vi "ReadLimits.vi"(8 "error in (no error)":errorcluster, 11 "PMUConfig":T1={"Class"="M", "Fs"=50.0, "F0"=50.0}) -> (0 "error out":errorcluster, 3 "Limits":dbl[][](array[numeric])=[[1.0, 1.0, 1.0, 1.0, 1.0, 1.0, 1.0, 1.0, 0.005, 0.1], [1.0, 1.0, 1.0, 1.0, 1.0, 1.0, 1.0, 1.0, inf, inf], [1.0, 1.0, 1.0, 1.0, 1.0, 1.0, 1.0, 1.0, 0.025, inf], [1.3, 1.3, 1.3, 1.3, 1.3, 1.3, 1.3, 1.3, 0.01, inf], [1.0, 1.0, 1.0, 1.0, 1.0, 1.0, 1.0, 1.0, 0.01, 0.2], [1.0, 1.0, 1.0, 1.0, 1.0, 1.0, 1.0, 1.0, 0.01, 0.2], [3.0, 3.0, 3.0, 3.0, 3.0, 3.0, 3.0, 3.0, 0.3, 14.0], [3.0, 3.0, 3.0, 3.0, 3.0, 3.0, 3.0, 3.0, 0.3, 14.0], [0.14, 0.14, 0.14, 0.14, 0.14, 0.14, 0.14, 0.14, 0.28, 0.28], [0.005, 0.005, 0.005, 0.005, 0.005, 0.005, 0.005, 0.005, inf, inf], [0.1, 0.1, 0.1, 0.1, 0.1, 0.1, 0.1, 0.1, inf, inf], [0.14, 0.14, 0.14, 0.14, 0.14, 0.14, 0.14, 0.14, 0.28, 0.28], [0.005, 0.005, 0.005, 0.005, 0.005, 0.005, 0.005, 0.005, inf, inf], [inf, inf, inf, inf, inf, inf, inf, inf, inf, inf]])   [LabVIEW 2014]
uses:
  typedef/PMUConfig.ctl
  typedef/ctlLimits.ctl
  typedef/clRptSS.ctl
  typedef/clTveFeRFe.ctl
  typedef/clRptRamp.ctl
  typedef/clRptMod.ctl
  typedef/clRptStep.ctl
  typedef/clStepVals.ctl
  <vilib>/Utility/xml.llb/Read From XML File(string).vi
panel:
  # "VA TVE"
  # "VB TVE"
  # "VC TVE"
  # "V+ TVE"
  # "IA TVE"
  # "IB TVE"
  # "IC TVE"
  # "I+ TVE"
  # "FE"
  # "RFE"
  # "FreqRng"
  # "MagRng"
  # "Harm"
  # "OOB"
  # "Phase Mod"
  # "Ampl Mod"
  # "Ramp +"
  # "Ramp -"
  # "Phase Step Response Time"
  # "Phase Step Delay Time"
  # "Phase Step Overshoot"
  # "Mag Step Response Time"
  # "Mag Step Delay Time"
  # "Mag Step Overshoot"
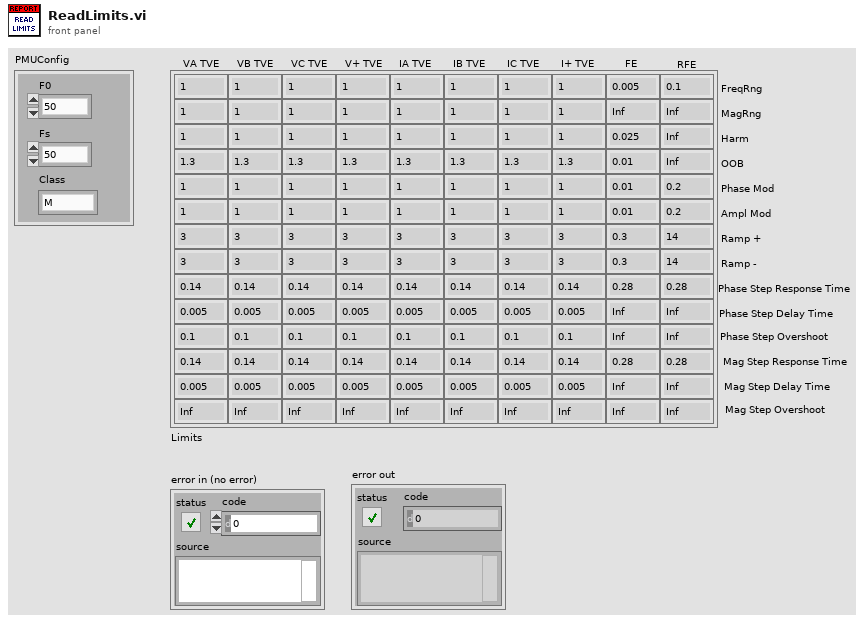
[diagram p1: front panel]
types:
  T1 = typedef "PMUConfig.ctl" = cluster{"Class":string, "Fs":dbl, "F0":dbl}
  T2 = typedef "ctlLimits.ctl" = cluster{"SteadyState":T3, "Ramp":T5, "Modulation":T6, "Step":T7, "Latency Test Limits":cluster{"Latency Limits":cluster{"Min Latency limit":dbl, "Max Latency limit":dbl}}}
  T3 = typedef "clRptSS.ctl" = cluster{"FreqResp":T4, "Harmonics":T4, "InterHarmonics":T4, "Mag":T4}
  T4 = typedef "clTveFeRFe.ctl" = cluster{"TVE":dbl, "Fe":dbl, "RFe":dbl}
  T5 = typedef "clRptRamp.ctl" = cluster{"ramp":T4}
  T6 = typedef "clRptMod.ctl" = cluster{"Phase":T4, "Amplitude":T4, "Combined":T4}
  T7 = typedef "clRptStep.ctl" = cluster{"Phase":T8, "Amplitude":T8}
  T8 = typedef "clStepVals.ctl" = cluster{"PhasorRespTime":dbl, "PhasorDelayTime":dbl, "PhaseOvershoot":dbl, "FreqRespTime":dbl, "ROCOFRespTime":dbl, "FreqOverShoot":dbl, "ROCOFOvershoot":dbl, "AmplOvershoot":dbl}
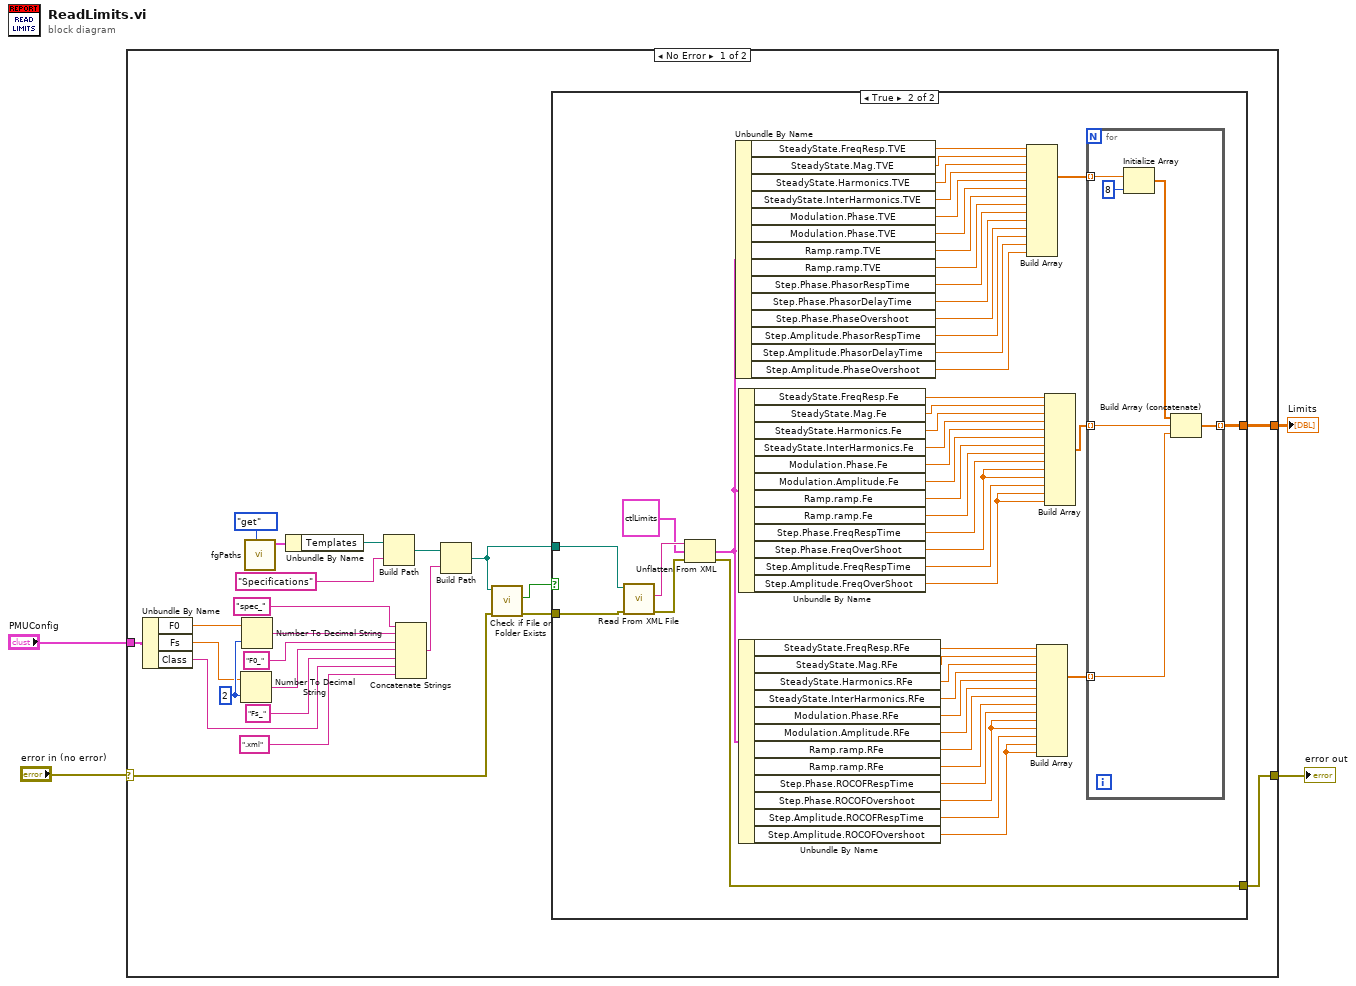
[diagram p0: block diagram]
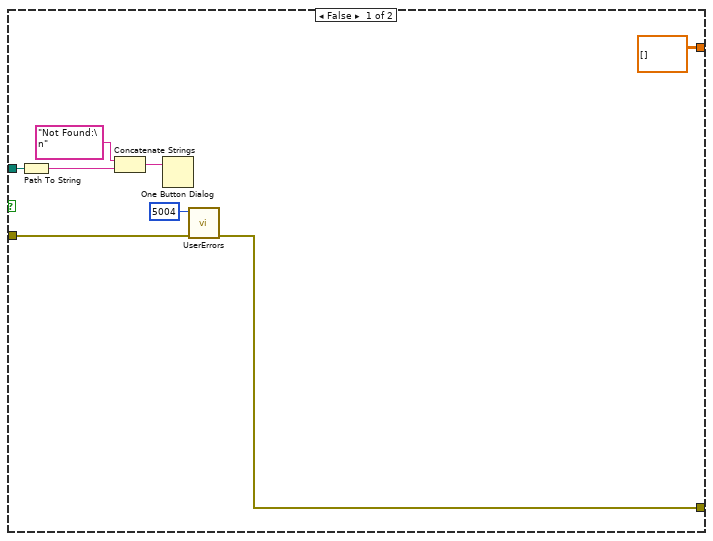
[diagram p2: hidden frame]
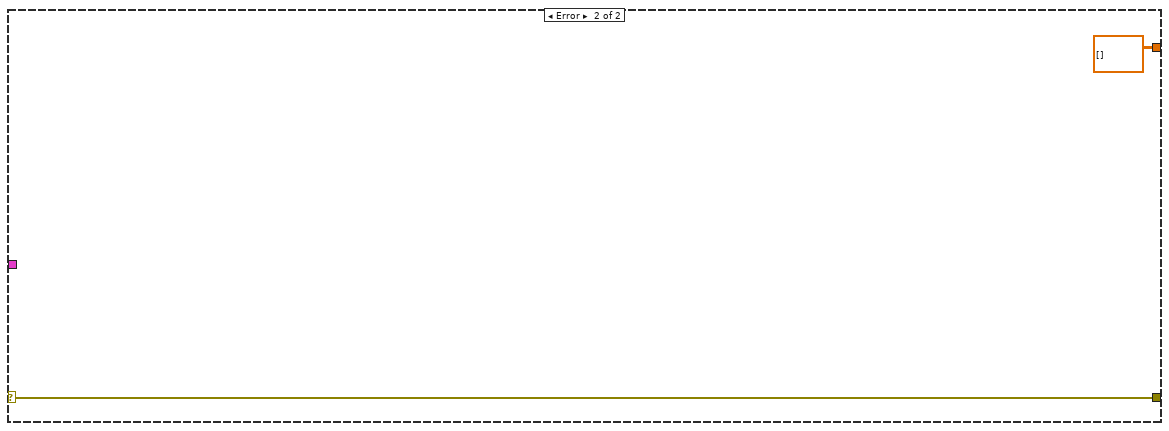
[diagram p3: hidden frame]
diagram:
  n1 = case shown="No Error" "error in (no error)" {
    selector: "error in (no error)" -> [w15 w92]
    tunnel: [w8 w92] -> w3
    tunnel: "PMUConfig" -> [w27 _]
    tunnel: [w9 dbl[][] []] -> w1
    frame No Error {
      w26 = i16 2 ("width (-)")
      n2 = Unbundle By Name(w27) -> ("F0"=w25:dbl, "Fs"=w24:dbl, "Class"=w11:string)
      n3 = Number To Decimal String(number=w24, width (-)=w26) -> (decimal integer string=w20:string)
      n4 = Number To Decimal String(number=w25, width (-)=w26) -> (decimal integer string=w22:string)
      n5 = call "fgPaths.vi"("cmd"=enum16{"init", "set", "get"}."get") -> ("clPaths"=w6:cluster{"Templates":path, "Reports":path})  [unwired: 9 in, 1 out]
      n6 = Unbundle By Name(w6) -> ("Templates"=w5:path)
      n7 = Build Path(base path=w5, name or relative path="Specifications") -> (appended path=w16:path)
      n8 = Concatenate Strings("spec_", w22, "F0_", w20, "Fs_", w11, ".xml") -> (w17:string)
      n9 = Build Path(base path=w16, name or relative path=w17) -> (appended path=w13:path)
      n10 = call <vilib>:"Check if File or Folder Exists.vi"("error in (no error)"=w15, "path"=w13) -> ("error out"=w14:errorcluster, "file or folder exists?"=w10:bool)  [unwired: 7 in, 1 out]
      n11 = case shown="True" w10 {
        tunnel: w14 -> [w35 w84]
        tunnel: w13 -> [w30 w83]
        tunnel: [w34 w50] -> w8
        tunnel: [dbl[][] [] w51] -> w9
        frame False {
          n12 = Path To String(path=w30) -> (string=w29:string)
          n13 = Concatenate Strings("Not Found:\n", w29) -> (w28:string)
          n14 = One Button Dialog(message=w28) -> ()  [unwired: 1 in, 1 out]
          n15 = call "UserErrors.vi"("error in (no error)"=w35, "[error code] (0)"=5004) -> ("error out"=w34:errorcluster)  [unwired: 9 in]
        }
        frame True {
          n16 = call-poly <vilib>:"Read From XML File.vi"("error in (no error)"=w84, "XML File Path"=w83) -> ("error out"=w81:errorcluster, "XML Elements"=w82:string)  [unwired: 7 in, 1 out]
          n17 = Unflatten From XML(xml string=w82, type=T2 {"SteadyState"={"FreqResp"={"TVE"=-inf, "Fe"=-inf, "RFe"=-inf}, "Harmonics"={"TVE"=-inf, "Fe"=-inf, "RFe"=-inf}, "InterHarmonics"={"TVE"=-inf, "Fe"=-inf, "RFe"=-inf}, "Mag"={"TVE"=-inf, "Fe"=-inf, "RFe"=-inf}}, "Ramp"={"ramp"={"TVE"=-inf, "Fe"=-inf, "RFe"=-inf}}, "Modulation"={"Phase"={"TVE"=-inf, "Fe"=-inf, "RFe"=-inf}, "Amplitude"={"TVE"=-inf, "Fe"=-inf, "RFe"=-inf}, "Combined"={"TVE"=-inf, "Fe"=-inf, "RFe"=-inf}}, "Step"={"Phase"={"PhasorRespTime"=-inf, "PhasorDelayTime"=-inf, "PhaseOvershoot"=-inf, "FreqRespTime"=-inf, "ROCOFRespTime"=-inf, "FreqOverShoot"=-inf, "ROCOFOvershoot"=-inf, "AmplOvershoot"=-inf}, "Amplitude"={"PhasorRespTime"=-inf, "PhasorDelayTime"=-inf, "PhaseOvershoot"=-inf, "FreqRespTime"=-inf, "ROCOFRespTime"=-inf, "FreqOverShoot"=-inf, "ROCOFOvershoot"=-inf, "AmplOvershoot"=-inf}}, "Latency Test Limits"={"Latency Limits"={"Min Latency limit"=0.0, "Max Latency limit"=0.0}}} ("ctlLimits"), error in (no error)=w81) -> (value=w61:T2, error out=w50:errorcluster)
          n18 = Unbundle By Name(w61) -> ("SteadyState.FreqResp.TVE"=w79:dbl, "SteadyState.Mag.TVE"=w78:dbl, "SteadyState.Harmonics.TVE"=w77:dbl, "SteadyState.InterHarmonics.TVE"=w76:dbl, "Modulation.Phase.TVE"=w75:dbl, "Modulation.Phase.TVE"=w74:dbl, "Ramp.ramp.TVE"=w73:dbl, "Ramp.ramp.TVE"=w71:dbl, "Step.Phase.PhasorRespTime"=w49:dbl, "Step.Phase.PhasorDelayTime"=w48:dbl, "Step.Phase.PhaseOvershoot"=w47:dbl, "Step.Amplitude.PhasorRespTime"=w46:dbl, "Step.Amplitude.PhasorDelayTime"=w45:dbl, "Step.Amplitude.PhaseOvershoot"=w44:dbl)
          n19 = Unbundle By Name(w61) -> ("SteadyState.FreqResp.Fe"=w70:dbl, "SteadyState.Mag.Fe"=w69:dbl, "SteadyState.Harmonics.Fe"=w68:dbl, "SteadyState.InterHarmonics.Fe"=w67:dbl, "Modulation.Phase.Fe"=w66:dbl, "Modulation.Amplitude.Fe"=w65:dbl, "Ramp.ramp.Fe"=w64:dbl, "Ramp.ramp.Fe"=w63:dbl, "Step.Phase.FreqRespTime"=w39:dbl, "Step.Phase.FreqOverShoot"=w38:dbl, "Step.Amplitude.FreqRespTime"=w37:dbl, "Step.Amplitude.FreqOverShoot"=w36:dbl)
          n20 = Unbundle By Name(w61) -> ("SteadyState.FreqResp.RFe"=w60:dbl, "SteadyState.Mag.RFe"=w59:dbl, "SteadyState.Harmonics.RFe"=w58:dbl, "SteadyState.InterHarmonics.RFe"=w57:dbl, "Modulation.Phase.RFe"=w56:dbl, "Modulation.Amplitude.RFe"=w55:dbl, "Ramp.ramp.RFe"=w54:dbl, "Ramp.ramp.RFe"=w53:dbl, "Step.Phase.ROCOFRespTime"=w43:dbl, "Step.Phase.ROCOFOvershoot"=w42:dbl, "Step.Amplitude.ROCOFRespTime"=w41:dbl, "Step.Amplitude.ROCOFOvershoot"=w40:dbl)
          n21 = Build Array(w79, w78, w77, w76, w75, w74, w73, w71, w49, w48, w47, w46, w45, w44) -> (w72:dbl[])
          n22 = Build Array(w60, w59, w58, w57, w56, w55, w54, w53, w43, w42, w42, w41, w40, w40) -> (w52:dbl[])
          n23 = Build Array(w70, w69, w68, w67, w66, w65, w64, w63, w39, w38, w38, w37, w36, w36) -> (w62:dbl[])
          n24 = for {
            tunnel: w72 -> [w90] mode=indexing
            tunnel: w62 -> [w87] mode=indexing
            tunnel: w52 -> [w86] mode=indexing
            tunnel: [w85] -> w51 mode=indexing
            n25 = Initialize Array(w90, 8 ("dimension size")) -> (w88:dbl[])
            n26 = Build Array (concatenate)(w88, w87, w86) -> (w85:dbl[])
          }
        }
      }
    }
    frame Error {
    }
  }
  "error out" <- w3
  "Limits" <- w1
